vi "ICC4C_Analog_Control_Tester_CHNL1_From_CSV_Importer_Template.vi"() -> ()   [LabVIEW 2021]
uses:
  <vilib>/DAQmx/write.llb/DAQmx Write (Analog 1D DBL NChan 1Samp).vi
  <vilib>/DAQmx/create/channels.llb/DAQmx Create Channel (AO-Voltage-Basic).vi
  <vilib>/DAQmx/miscellaneous.llb/DAQmx Fill In Error Info.vi
panel:
  out "ICC4C 01":dbl
  out "current mA":dbl
  in  "mA Step Size":dbl
  in  "Y1 (-10-10V)":dbl
  in  "X1 (-10-10V)":dbl
  out "Raw  Inner Loop Iternation":i32
  out "Andor_V":dbl
  out "Trigger_Phase_Iterations":i32
  in  "Delay (ADDS 3ms)":i32
  in  "ICC4C 3 (0-10V)":dbl
  in  "ICC4C 2 (0-10V)":dbl
  in  "ICC4C 0 (0-10V)":dbl
  in  "Y2 (-10-10V)":dbl
  in  "X2 (-10-10V)":dbl
  in  "Continue Cycle?":bool
  out "Full Cycles":i32
  out "Mirror_Phase_Iterations":i32
  in  "Blanking (0-10v)":dbl=10.0
  in  "561 (0-10v)":dbl
  in  "514 (0-10v)":dbl
  in  "488 (0-10v)":dbl
  in  "445 (0-10v)":dbl
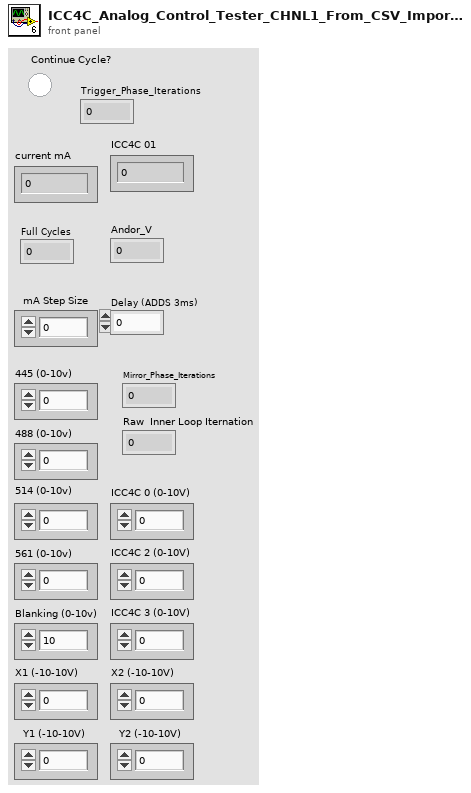
[diagram p1: front panel]
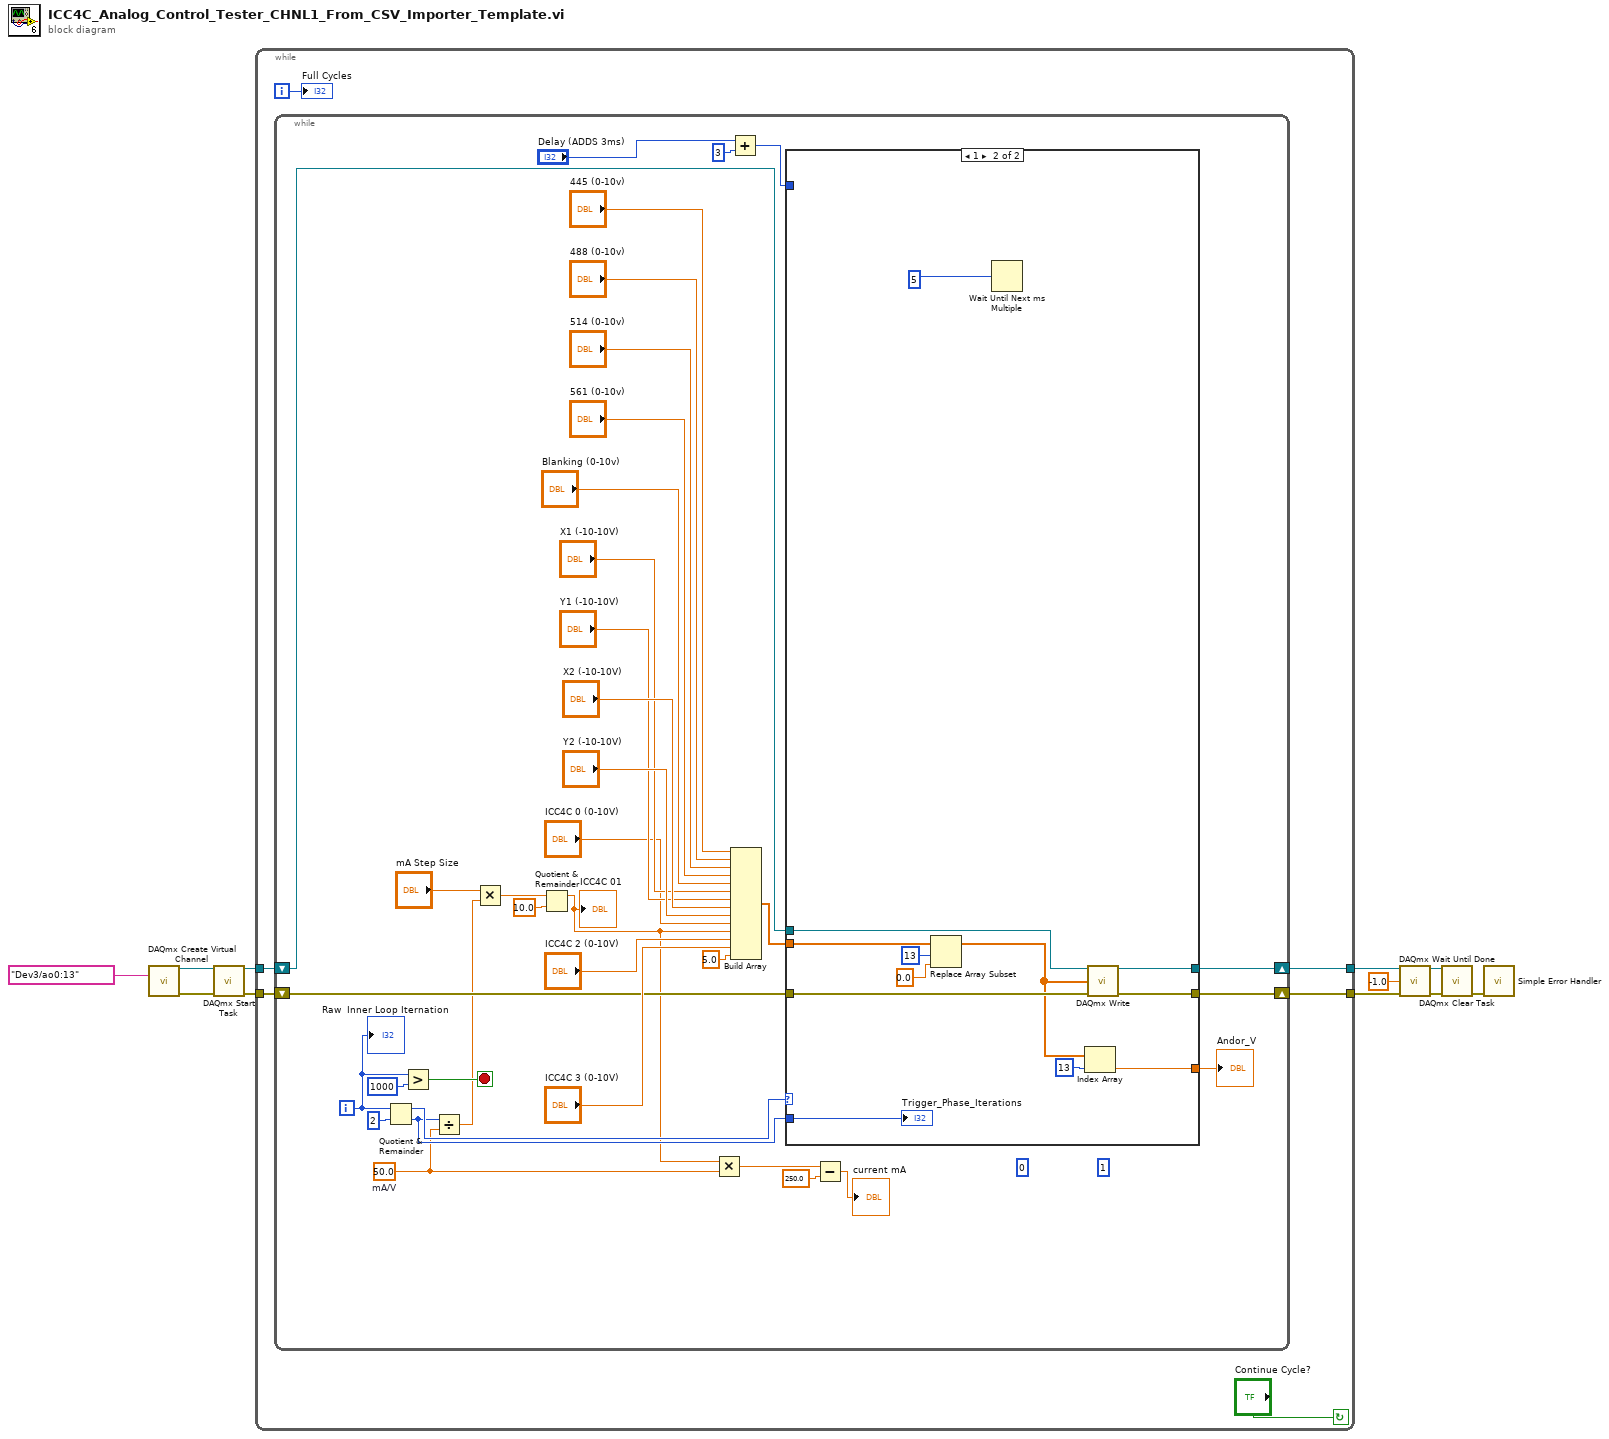
[diagram p0: block diagram]
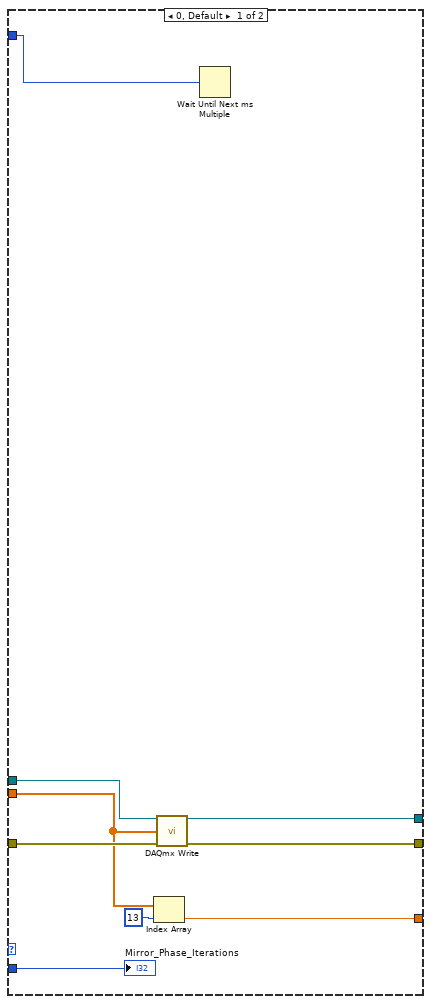
[diagram p2: hidden frame]
diagram:
  n1 = call-poly <vilib>:"DAQmx Create Virtual Channel.vi"("physical channels"=tag "Dev3/ao0:13") -> ("task out"=w4:refnum<k21>, "error out"=w3:errorcluster)  [unwired: 13 in]
  n2 = call <vilib>:"DAQmx Start Task.vi"("task/channels in"=w4, "error in"=w3) -> ("task out"=w2:refnum<k21>, "error out"=w1:errorcluster)  [unwired: 12 in]
  n3 = while {
    tunnel: [w14] -> w7
    tunnel: [w13] -> w6
    tunnel: w2 -> [w16]
    tunnel: w1 -> [w15]
    i -> [w17]
    stop <- "Continue Cycle?" continue-if-true
    n4 = while {
      shift-right: [w43] -> w14
      shift-left: w16 -> [w41]
      shift-right: [w44] -> w13
      shift-left: w15 -> [w40]
      i -> [w33]
      stop <- w31 stop-if-true
      w23 = 50.0  # mA/V
      (unwired) 0
      (unwired) 1
      n5 = Quotient & Remainder(x=w33, y=2) -> (x-y*floor(x/y)=w34:i32, floor(x/y)=w29:i32)
      n6 = Greater?(x=w33, y=1000) -> (0:w31:bool)
      n7 = Divide(x=w29, y=w23) -> (x/y=w28:dbl)
      n8 = Multiply(x="mA Step Size", y=w28) -> (x*y=w25:dbl)
      n9 = Quotient & Remainder(x=w25, y=10.0) -> (x-y*floor(x/y)=w19:dbl)  [unwired: 1 out]
      "ICC4C 01" <- w19
      n10 = Multiply(x=w19, y=w23) -> (x*y=w22:dbl)
      n11 = Add(x="Delay (ADDS 3ms)", y=3) -> (x+y=w18:i32)
      n12 = Build Array("445 (0-10v)", "488 (0-10v)", "514 (0-10v)", "561 (0-10v)", "Blanking (0-10v)", "X1 (-10-10V)", "Y1 (-10-10V)", "X2 (-10-10V)", "Y2 (-10-10V)", "ICC4C 0 (0-10V)", w19, "ICC4C 2 (0-10V)", "ICC4C 3 (0-10V)", 5.0) -> (w45:dbl[])
      n13 = case shown="1" w34 {
        tunnel: w41 -> [w63 w75]
        tunnel: [w60 w74] -> w43
        tunnel: w40 -> [w62 w73]
        tunnel: [w61 w69] -> w44
        tunnel: w45 -> [w59 w72]
        tunnel: w29 -> [w56 w70]
        tunnel: [w57 w66] -> w39
        tunnel: w18 -> [w55 _]
        frame 0, Default {
          n14 = Index Array(array=w59, index=13) -> (element=w57:dbl)
          n15 = call-poly <vilib>:"DAQmx Write.vi"("task/channels in"=w63, "data"=w59, "error in"=w62) -> ("task out"=w60:refnum<k21>, "error out"=w61:errorcluster)  [unwired: 10 in, 1 out]
          n16 = Wait Until Next ms Multiple(millisecond multiple=w55) -> ()  [unwired: 1 out]
          "Mirror_Phase_Iterations" <- w56
        }
        frame 1 {
          n17 = Replace Array Subset(array=w72, new element=0.0, index=13) -> (w67:dbl[])
          n18 = Wait Until Next ms Multiple(millisecond multiple=5) -> ()  [unwired: 1 out]
          n19 = Index Array(array=w67, index=13) -> (element=w66:dbl)
          n20 = call-poly <vilib>:"DAQmx Write.vi"("task/channels in"=w75, "data"=w67, "error in"=w73) -> ("task out"=w74:refnum<k21>, "error out"=w69:errorcluster)  [unwired: 10 in, 1 out]
          "Trigger_Phase_Iterations" <- w70
        }
      }
      "Andor_V" <- w39
      n21 = Subtract(x=w22, y=250.0) -> (x-y=→"current mA":dbl)
      "Raw  Inner Loop Iternation" <- w33
    }
    "Full Cycles" <- w17
  }
  n22 = call <vilib>:"DAQmx Wait Until Done.vi"("task/channels in"=w7, "timeout (sec)"=-1.0, "error in"=w6) -> ("task out"=w10:refnum<k21>, "error out"=w9:errorcluster)  [unwired: 11 in]
  n23 = call <vilib>:"DAQmx Clear Task.vi"("task in"=w10, "error in"=w9) -> ("error out"=w11:errorcluster)  [unwired: 13 in]
  n24 = call <vilib>:"Simple Error Handler.vi"("error in (no error)"=w11) -> ()  [unwired: 4 in, 5 out]
